vi "ArrDevMeasAction.vi"(7 "DevId":i32, 8 "error in (no error)":errorcluster caption="entrée d'erreur (pas d'erreur)", 9 "CurvePointIndex":i32, 10 "AllPointIndex":i32, 11 "Device In":refnum<class "MultiHarp150.lvclass"> caption="DNL_LabVIEW Object in") -> (0 "error out":errorcluster caption="sortie d'erreur", 1 "ArrDevDat":T1[](array[typedef]), 2 "ArrDevDatOut":dbl[][](array[numeric]), 3 "Device Out":refnum<class "MultiHarp150.lvclass"> caption="DNL_LabVIEW Object out", 5 "MeasOut":dbl[](array[numeric]))   [LabVIEW 2019, in "MultiHarp150.lvclass"]
uses:
  MultiHarp150.lvclass
  C:/Programmes Labview/LabscanV1A/DevicesClass/BaseDevice/BaseDevice.lvclass
  Experiment Class/ArrDevData.ctl
  MultiHarp150.lvclass/MultiHarp150.ctl
  <userlib>/MultiHarp150/T2Lib/MH_T2QMessage.ctl
  T2AcqStates.ctl
  <userlib>/GenProg/ReadValByRefI32.vi
  <vilib>/Utility/error.llb/Error Cluster From Error Code.vi
  <vilib>/ErrorRing/Error Ring.xnode
panel:
  out "TotalT":u32
  out "Desired LP":u32[](array[numeric])
  out "Loop DeltaT":u32[](array[numeric])
  out "RecRate":u32
  out "LoopPeriod":u32
  out "Record/ms":dbl
  in  "RecordsCnt":i64
  in  "OverRun":bool
  in  "Acq":bool
  out "Graph":refnum<vi>
  out "Dat":refnum<vi>
  in  "ViRef":refnum<vi>
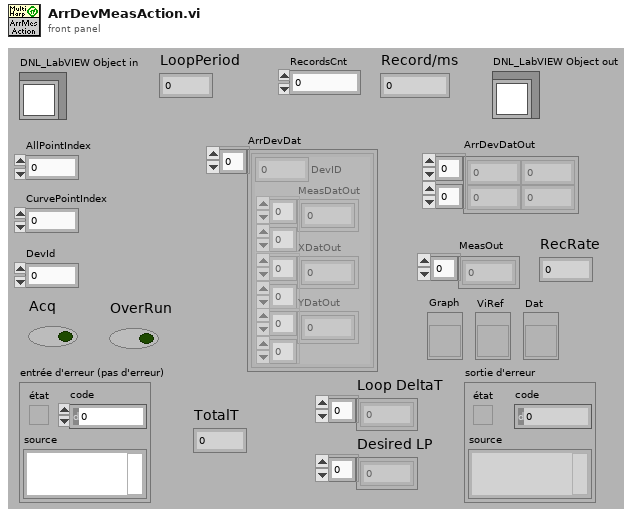
[diagram p1: front panel]
types:
  T1 = typedef "ArrDevData.ctl" = cluster{"MeasDatOut":dbl[][], "XDatOut":dbl[][], "YDatOut":dbl[][], "DevID":i32}
  T2 = cluster{"TotalCount":dbl, "HistRate (CPS)":dbl, "MaxTime":dbl}[]
  T3 = enum32{"Invalid", "Standard", "Closed", "Hidden", "Minimized", "Maximized"}
  T4 = typedef "T2AcqStates.ctl" = enum16{"checkStatus", "ReadFifo", "StopMeas", "Error", "End"}
  T5 = typedef "MH_T2QMessage.ctl" = cluster{"Message":string, "buffer":u32[], "Code":i32, "nactual":i32}
  T6 = typedef "MH_InputChannel_LS.ctl" = cluster{"Name":string, "Enable":bool, "Edge":i32, "Level":i32, "Offset":i32, "UseDeadTime":bool, "DeadTime":i32}
  T7 = typedef "MultiHarp150.lvclass/MultiHarp150_Func.ctl" = enum16{"ReadHistogram (Ph)", "ReadT2 (Ph)", "ReadT3 (Ph)", "ReadCount (Ph)"}
  T8 = cluster{dbl, "Resolution (ns)":dbl, "Histogram":u32[][]}
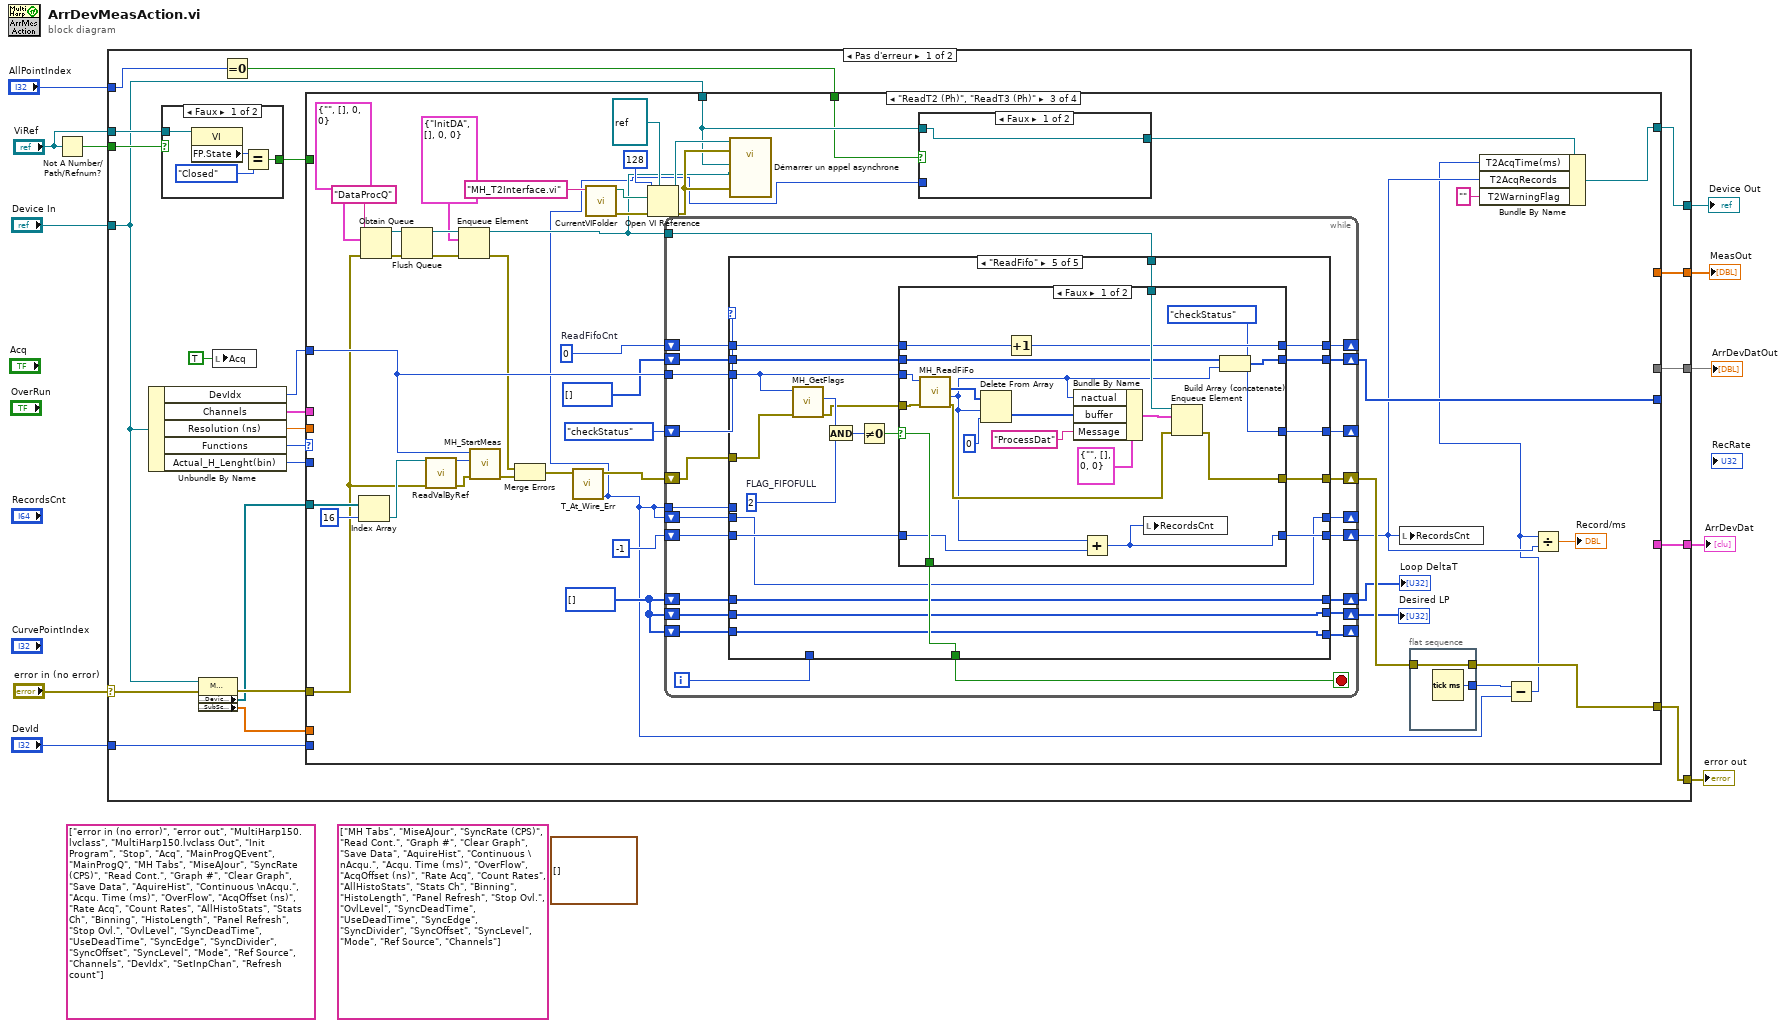
[diagram p0: block diagram]
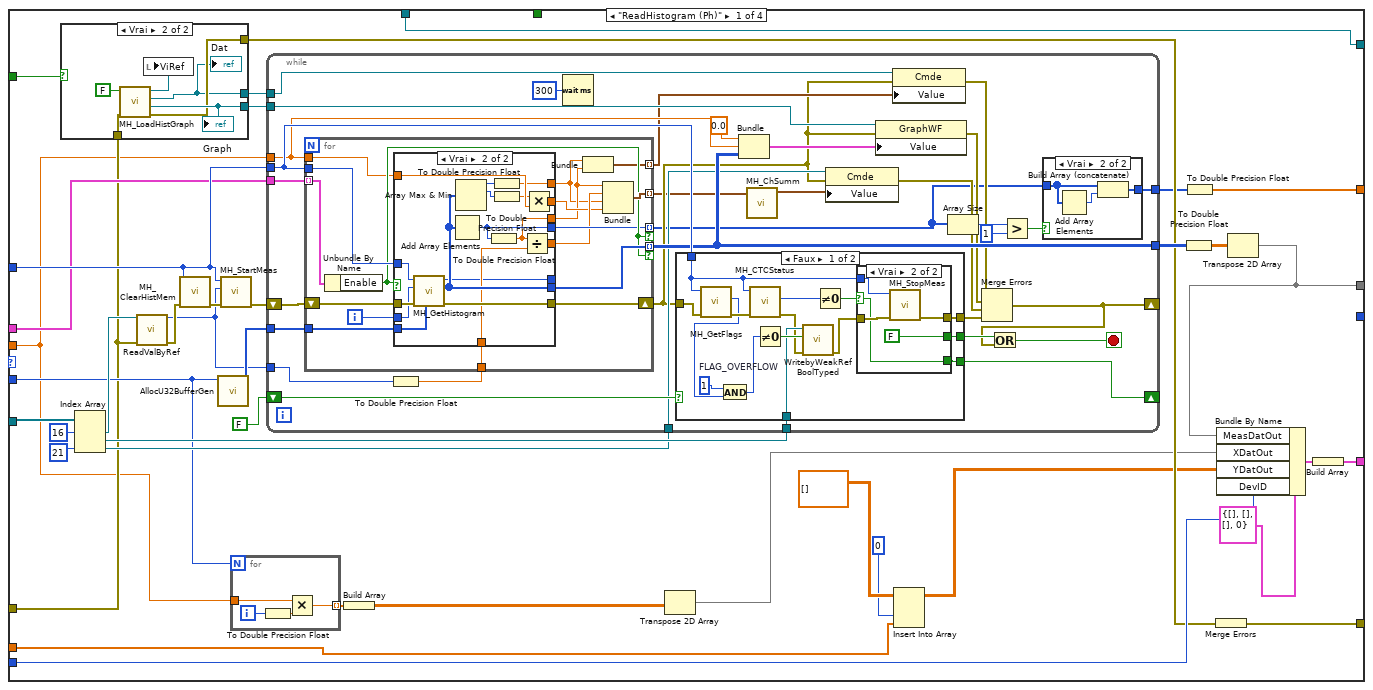
[diagram p3: hidden frame]
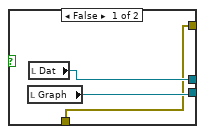
[diagram p4: hidden frame]
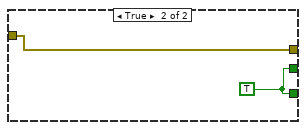
[diagram p7: hidden frame]
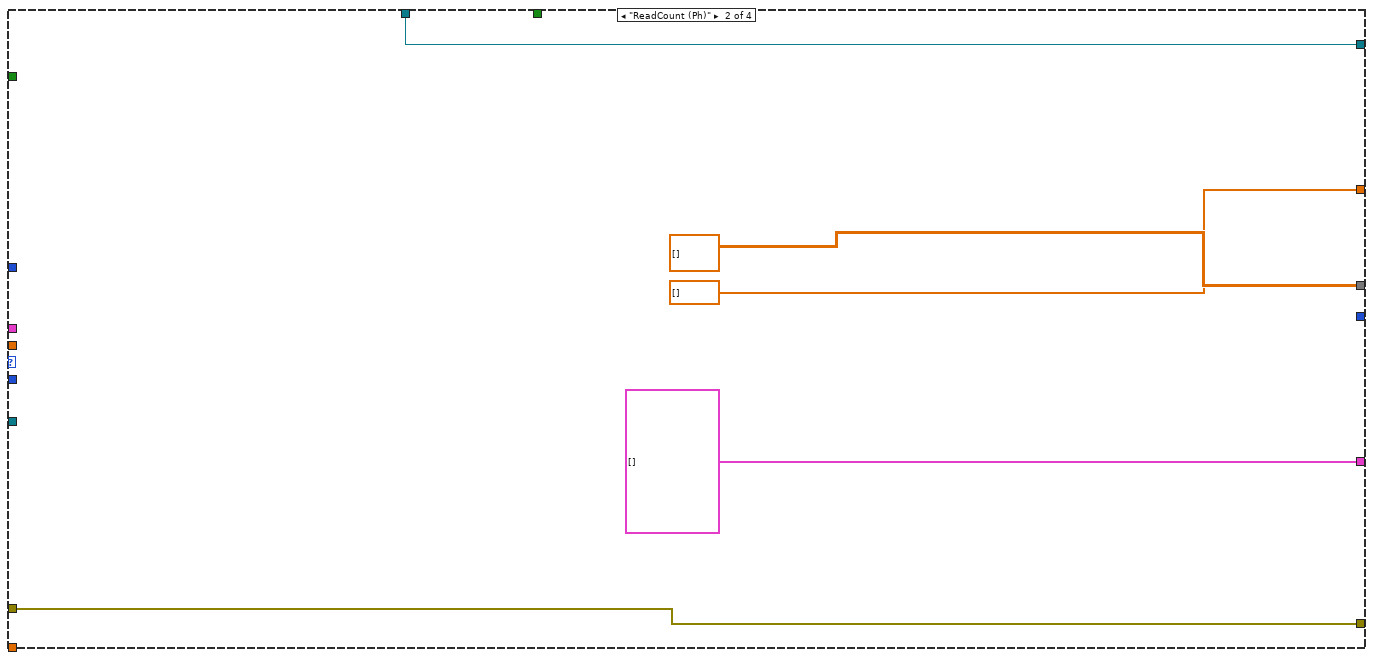
[diagram p9: hidden frame]
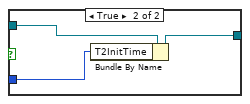
[diagram p10: hidden frame]
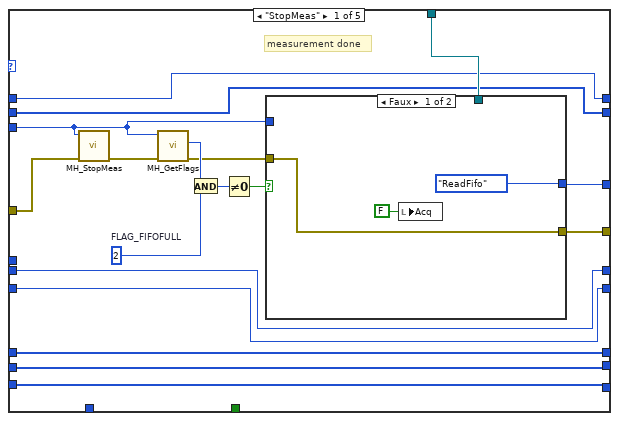
[diagram p11: hidden frame]
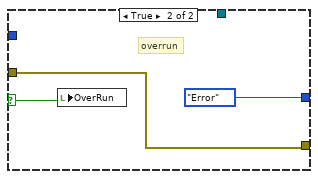
[diagram p12: hidden frame]
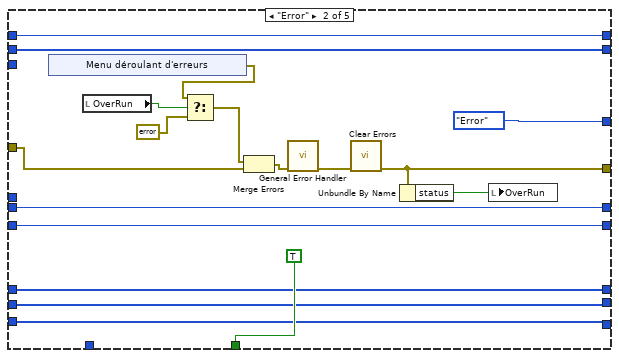
[diagram p13: hidden frame]
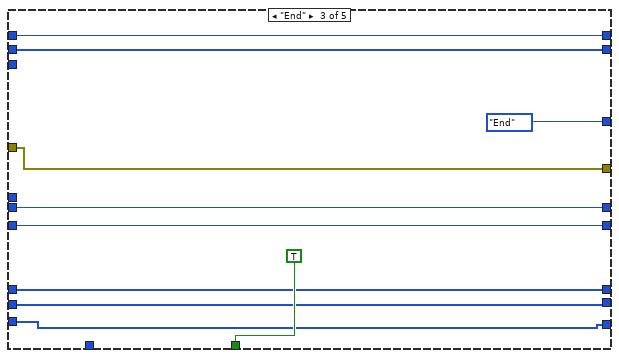
[diagram p14: hidden frame]
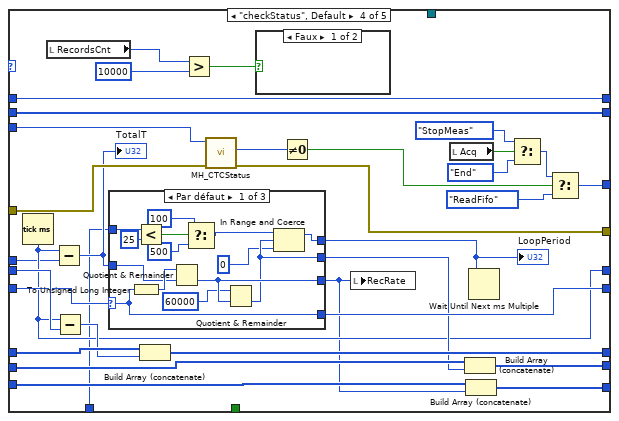
[diagram p15: hidden frame]
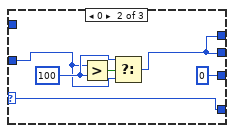
[diagram p16: hidden frame]
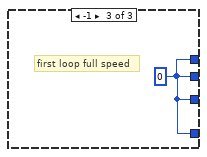
[diagram p17: hidden frame]
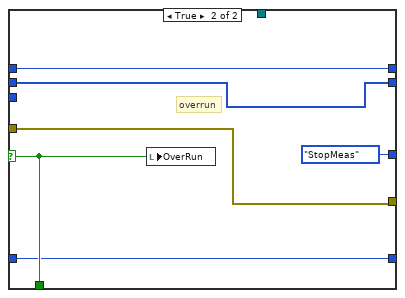
[diagram p19: hidden frame]
diagram:
  (unwired) string[][] [["MH Tabs"], ["MiseAJour"], ["SyncRate (CPS)"], ["Read Cont."], ["Graph #"], ["Clear Graph"], ["Save Data"], ["AquireHist"], ["Continuous \nAcqu."], ["Acqu. Time (ms)"], ["OverFlow"], ["AcqOffset (ns)"], ["Rate Acq"], ["Count Rates"], ["AllHistoStats"], ["Stats Ch"], ["Binning"], ["HistoLength"], ["Panel Refresh"], ["Stop Ovl."], ["OvlLevel"], ["SyncDeadTime"], ["UseDeadTime"], ["SyncEdge"], ["SyncDivider"], ["SyncOffset"], ["SyncLevel"], ["Mode"], ["Ref Source"], ["Channels"]] ("TabControls")
  (unwired) string[] ["error in (no error)", "error out", "MultiHarp150.lvclass", "MultiHarp150.lvclass Out", "Init Program", "Stop", "Acq", "MainProgQEvent", "MainProgQ", "MH Tabs", "MiseAJour", "SyncRate (CPS)", "Read Cont.", "Graph #", "Clear Graph", "Save Data", "AquireHist", "Continuous \nAcqu.", "Acqu. Time (ms)", "OverFlow", "AcqOffset (ns)", "Rate Acq", "Count Rates", "AllHistoStats", "Stats Ch", "Binning", "HistoLength", "Panel Refresh", "Stop Ovl.", "OvlLevel", "SyncDeadTime", "UseDeadTime", "SyncEdge", "SyncDivider", "SyncOffset", "SyncLevel", "Mode", "Ref Source", "Channels", "DevIdx", "SetInpChan", "Refresh count"] ("ControlsNames")
  (unwired) T2 [] ("AllHistoStats")
  n1 = Not A Number/Path/Refnum?(number/path/refnum="ViRef") -> (NaN/Path/Refnum?=w2:bool)
  n2 = case shown="Pas d'erreur" "error in (no error)" {
    selector: "error in (no error)" -> [w31 w431]
    tunnel: [w32 w431] -> w10
    tunnel: [w14 w430] -> w9
    tunnel: "Device In" -> [w15 w430]
    tunnel: "AllPointIndex" -> [w13 _]
    tunnel: [w28 dbl[] [] ("MeasOut 2")] -> w6
    tunnel: [w27 dbl[][] [] ("ArrDevDatOut 2")] -> w5
    tunnel: [w25 T1[] [] ("ArrDevDat 2")] -> w4
    tunnel: "DevId" -> [w26 _]
    tunnel: w2 -> [w17 _]
    tunnel: "ViRef" -> [w19 _]
    frame No Error {
      n3 = Unbundle By Name(w15) -> ("DevIdx"=w21:i32, "Channels"=w22:T6[], "Resolution (ns)"=w24:dbl, "Functions"=w33:T7, "Actual_H_Lenght(bin)"=w23:i32)
      n4 = case shown="Faux" w17 {
        selector: w17 -> [_ w38]
        tunnel: w19 -> [w37 _]
        tunnel: [w34 w38] -> w18
        frame False {
          n5 = property class="VI"(reference=w37) -> ("FP.State"=w36:T3)  [unwired: 1 in, 2 out]
          n6 = Equal?(x=w36, y=T3."Closed") -> (x = y?=w34:bool)
        }
        frame True {
        }
      }
      n7 = property class="MultiHarp150.lvclass"(reference=w15, error in=w31) -> (error out=w30:errorcluster, "Accessor:DeviceCtrl"=w29:refnum<vi>[], "Accessor:SubScanTable(y)"=w20:dbl[])  [unwired: 1 out]
      n8 = local write "Acq"(TRUE ("Acq")) -> ()
      n9 = Equal To 0?(x=w13) -> (x = 0?=w12:bool)
      n10 = case shown="\"ReadT2 (Ph)\", \"ReadT3 (Ph)\"" w33 {
        tunnel: [w65 w188 w217 w426] -> w32
        tunnel: w30 -> [w52 w188 w226 w426]
        tunnel: w29 -> [w53 _ w236 _]
        tunnel: [w69 dbl[] [] _ _] -> w28
        tunnel: [w46 dbl[][] [] _ _] -> w27
        tunnel: w26 -> [w74 _ _ _]
        tunnel: [w72 T1[] [] _ _] -> w25
        tunnel: w21 -> [w61 _ w231 _]
        tunnel: w24 -> [w45 _ _ _]
        tunnel: w23 -> [w55 _ _ _]
        tunnel: w22 -> [w56 _ _ _]
        tunnel: w20 -> [w54 _ _ _]
        tunnel: w18 -> [w43 _ _ _]
        tunnel: [_ _ w212 _] -> _
        tunnel: w15 -> [w39 w187 w194 w425]
        tunnel: [w39 w187 w201 w425] -> w14
        tunnel: w12 -> [_ _ w193 _]
        frame "ReadHistogram (Ph)" {
          n11 = case shown="Vrai" w43 {
            tunnel: [w80 w86] -> w63
            tunnel: [w78 w85] -> w62
            tunnel: w52 -> [w78 w84]
            tunnel: [w79 w83] -> w44
            frame False {
              n12 = local read "Graph"() -> (w80:refnum<vi>)
              n13 = local read "Dat"() -> (w79:refnum<vi>)
            }
            frame True {
              n14 = call <userlib>:"MH_LoadHistGraph.vi"("ErrIn(No Err)"=w84, "Rate Mode"=FALSE) -> ("ErrOut"=w85:errorcluster, "Graph"=w86:refnum<vi>, "Dat"=w83:refnum<vi>, "ViRef"=w82:refnum<vi>)  [unwired: 4 in, 2 out]
              "Dat" <- w83
              "Graph" <- w86
              n15 = local write "ViRef"(w82) -> ()
            }
          }
          n16 = Index Array(array=w53, index #1=16 ("indice"), index #3=21 ("indice")) -> (element #1=w76:refnum<vi>, element #2=w66:refnum<vi>, element #3=w57:refnum<vi>)  [unwired: 1 in]
          n17 = call-poly <userlib>:"ReadValByRef.vi"("Control Ref"=w76, "error in"=w52) -> ("Valeur"=w40:i32, "error out"=w67:errorcluster)  [unwired: 12 in]
          n18 = call <userlib>:"MH_ClearHistMem.vi"("error in (no error)"=w67, "devidx"=w61) -> ("error out"=w68:errorcluster)  [unwired: 8 in, 1 out]
          n19 = call <userlib>:"AllocU32BufferGen.vi"("BuffLength"=w55) -> ("Buffer"=w71:u32[])  [unwired: 10 in]
          n20 = call <userlib>:"MH_StartMeas.vi"("error in (no error)"=w68, "tacq"=w40, "devidx"=w61) -> ("error out"=w70:errorcluster)  [unwired: 7 in, 1 out]
          n21 = for {
            N: w55 -> [_]
            tunnel: w45 -> [w90]
            tunnel: [w87] -> w42 mode=indexing
            i -> [w89]
            n22 = To Double Precision Float(number=w89) -> (double precision float=w88:dbl)
            n23 = Multiply(x=w90, y=w88) -> (x*y=w87:dbl)
          }
          n24 = while {
            tunnel: w56 -> [w106]
            tunnel: [w117] -> w64
            tunnel: w61 -> [w120]
            shift-right: [w111] -> _
            shift-left: w70 -> [w122]
            tunnel: w71 -> [w123]
            tunnel: w66 -> [w119]
            tunnel: w45 -> [w105]
            tunnel: w63 -> [w115]
            shift-right: [w110] -> _
            shift-left: FALSE -> [w109]
            tunnel: [w95] -> w58
            tunnel: w57 -> [w108]
            tunnel: w40 -> [w107]
            tunnel: w44 -> [w104]
            stop <- w113 stop-if-true
            n25 = To Double Precision Float(number=w107) -> (double precision float=w93:dbl)
            n26 = for {
              tunnel: w123 -> [w168]
              tunnel: w120 -> [w167]
              tunnel: w106 -> [w164] mode=indexing
              shift-right: [w165] -> w101
              shift-left: w122 -> [w166]
              tunnel: [w163] -> w117 mode=indexing if=w161
              tunnel: [w159] -> w96 mode=indexing if=w161
              tunnel: w105 -> [w157]
              tunnel: [w162] -> w91 mode=indexing
              tunnel: w93 -> [w160]
              tunnel: [w156] -> w103 mode=indexing
              i -> [w154]
              n27 = Unbundle By Name(w164) -> ("Enable"=w161:bool)
              n28 = case shown="Vrai" w161 {
                tunnel: w168 -> [_ w186]
                tunnel: w167 -> [_ w175]
                tunnel: [_ w182] -> w163
                tunnel: w166 -> [w169 w185]
                tunnel: [w169 w184] -> w165
                tunnel: w154 -> [_ w183]
                tunnel: [_ w178] -> w159
                tunnel: w157 -> [_ w180]
                tunnel: [_ w179] -> w155
                tunnel: w160 -> [_ w177]
                tunnel: [_ w176] -> w158
                tunnel: [_ w174] -> _
                tunnel: [_ w173] -> w153
                tunnel: [_ w171] -> w152
                frame False {
                }
                frame True {
                  n29 = call <userlib>:"MH_GetHistogram.vi"("Chcount"=w186, "error in (no error)"=w185, "channel"=w183, "devidx"=w175) -> ("error out"=w184:errorcluster, "Histogram"=w182:u32[], "return type"=w174:i32)  [unwired: 5 in]
                  n30 = Add Array Elements(numeric array=w182) -> (sum=w178:u32)
                  n31 = Array Max & Min(array=w182) -> (max value=w172:u32, max index (indices)=w181:i32)  [unwired: 2 out]
                  n32 = To Double Precision Float(number=w178) -> (double precision float=w173:dbl)
                  n33 = To Double Precision Float(number=w172) -> (double precision float=w171:dbl)
                  n34 = To Double Precision Float(number=w181) -> (double precision float=w170:dbl)
                  n35 = Divide(x=w173, y=w177) -> (x/y=w176:dbl)
                  n36 = Multiply(x=w170, y=w180) -> (x*y=w179:dbl)
                }
              }
              n37 = Bundle(w152, w153) -> (w156:cluster{dbl, dbl})  [unwired: 1 in]
              n38 = Bundle(w153, w158, w152, w155) -> (w162:cluster{dbl, dbl, dbl, dbl})  [unwired: 1 in]
            }
            n39 = Wait (ms)(milliseconds to wait=u32 300 ("attente (ms)")) -> ()  [unwired: 1 out]
            n40 = case shown="Faux" w109 {
              tunnel: w101 -> [w136 w151]
              tunnel: [w131 w150] -> w121
              tunnel: w120 -> [w135 _]
              tunnel: w119 -> [w137 _]
              tunnel: [w133 w151] -> w112
              tunnel: [w130 w150] -> w110
              frame False {
                w140 = 1  # FLAG_OVERFLOW
                n41 = call <userlib>:"MH_GetFlags.vi"("error in (no error)"=w136, "devidx"=w135) -> ("error out"=w142:errorcluster, "flags"=w139:i32)  [unwired: 7 in, 1 out]
                n42 = And(x=w140, y=w139) -> (x .and. y?=w141:i32)
                n43 = call <userlib>:"MH_CTCStatus.vi"("error in (no error)"=w142, "devidx"=w135) -> ("error out"=w129:errorcluster, "ctcstatus"=w134:i32)  [unwired: 7 in, 1 out]
                n44 = Not Equal To 0?(x=w141) -> (x != 0?=w138:bool)
                n45 = call <userlib>:"WritebyWeakRefBoolTyped.vi"("error in"=w129, "Valeur"=w138, "Control Ref"=w137) -> ("error out"=w128:errorcluster)  [unwired: 8 in]
                n46 = Not Equal To 0?(x=w134) -> (x != 0?=w132:bool)
                n47 = case shown="Vrai" w132 {
                  selector: w132 -> [w143 w145]
                  tunnel: w135 -> [_ w147]
                  tunnel: w128 -> [w144 w149]
                  tunnel: [w144 w148] -> w133
                  tunnel: [w143 FALSE] -> w131
                  tunnel: [w143 w145] -> w130
                  frame False {
                  }
                  frame True {
                    n48 = call <userlib>:"MH_StopMeas.vi"("error in (no error)"=w149, "devidx"=w147) -> ("error out"=w148:errorcluster)  [unwired: 8 in, 1 out]
                  }
                }
              }
              frame True {
                w150 = TRUE
              }
            }
            n49 = Bundle(0.0, "Resolution (ns)"=w105, "Histogram"=w117) -> (w114:T8)  [unwired: 1 in]
            n50 = call <userlib>:"MH_ChSumm.vi"("HistDat"=w91) -> ("HistDat Out"=w92:cluster{dbl, dbl, dbl, dbl}[])  [unwired: 10 in]
            n51 = property class="Cmde"(reference=w108, error in=w101, "Value"=w92) -> (error out=w100:errorcluster)  [unwired: 1 out]
            n52 = property class="GraphWF"(reference=w115, error in=w101, "Value"=w114) -> (error out=w99:errorcluster)  [unwired: 1 out]
            n53 = property class="Cmde"(reference=w104, error in=w101, "Value"=w103) -> (error out=w102:errorcluster)  [unwired: 1 out]
            n54 = Array Size(array=w96) -> (size(s)=w98:i32)
            n55 = Merge Errors(w102, w99, w100, w112) -> (w111:errorcluster)
            n56 = Or(x=w121, y=w111) -> (x .or. y?=w113:bool)
            n57 = Greater?(x=w98, y=1) -> (0:w94:bool)
            n58 = case shown="Vrai" w94 {
              tunnel: w96 -> [w124 w126]
              tunnel: [w124 w125] -> w95
              frame False {
              }
              frame True {
                n59 = Add Array Elements(numeric array=w126) -> (sum=w127:u32)
                n60 = Build Array (concatenate)(w126, w127) -> (w125:u32[])
              }
            }
          }
          n61 = Build Array(w42) -> (w41:dbl[][])
          n62 = Transpose 2D Array(2D array=w41) -> (transposed array=w48:dbl[][])
          n63 = Insert Into Array(array=dbl[][] [] ("tableau"), index (col)=0 ("indice désactivé (col)"), new element=w54) -> (w51:dbl[][])  [unwired: 1 in]
          n64 = To Double Precision Float(number=w64) -> (double precision float=w47:dbl[][])
          n65 = To Double Precision Float(number=w58) -> (double precision float=w69:dbl[])
          n66 = Merge Errors(w62) -> (w65:errorcluster)
          n67 = Transpose 2D Array(2D array=w47) -> (transposed array=w46:dbl[][])
          n68 = Bundle By Name(cluster=T1 {"MeasDatOut"=[], "XDatOut"=[], "YDatOut"=[], "DevID"=0} ("cluster de sortie"), "MeasDatOut"=w46, "XDatOut"=w48, "YDatOut"=w51, "DevID"=w74) -> (w73:T1)
          n69 = Build Array(w73) -> (w72:T1[])
        }
        frame "ReadCount (Ph)" {
        }
        frame "ReadT2 (Ph)", "ReadT3 (Ph)" {
          w210 = u32[] []
          w221 = u32 0  # ReadFifoCnt
          n70 = Index Array(array=w236, index=16 ("indice")) -> (element=w235:refnum<vi>)
          n71 = Obtain Queue(name (unnamed)="DataProcQ", element data type=T5 {"Message"="", "buffer"=[], "Code"=0, "nactual"=0} ("ClassQueue"), error in (no error)=w226) -> (queue out=w230:refnum<queue>, error out=w229:errorcluster)  [unwired: 2 in, 1 out]
          n72 = Flush Queue(queue=w230, error in (no error)=w229) -> (queue out=w225:refnum<queue>, error out=w224:errorcluster)  [unwired: 1 out]
          n73 = call-poly <userlib>:"ReadValByRef.vi"("Control Ref"=w235, "error in"=w226) -> ("Valeur"=w234:i32, "error out"=w233:errorcluster)  [unwired: 12 in]
          n74 = Enqueue Element(queue=w225, element=T5 {"Message"="InitDA", "buffer"=[], "Code"=0, "nactual"=0} ("élément"), error in (no error)=w224) -> (queue out=w202:refnum<queue>, error out=w223:errorcluster)  [unwired: 1 in, 1 out]
          n75 = call <userlib>:"MH_StartMeas.vi"("error in (no error)"=w233, "tacq"=w234, "devidx"=w231) -> ("error out"=w232:errorcluster)  [unwired: 7 in, 1 out]
          n76 = Merge Errors(w223, w232) -> (w197:errorcluster)
          n77 = call <userlib>:"T_At_Wire_Err.vi"("error in (no error)"=w197) -> ("Clock(ms)"=w192:u32, "error out"=w196:errorcluster)  [unwired: 8 in, 1 out]
          n78 = call <userlib>:"CurrentVIFolder.vi"("NomFichier"="MH_T2Interface.vi" ("nom ou chemin relatif")) -> ("error out"=w205:errorcluster, "Chemin"=w204:path)  [unwired: 8 in, 1 out]
          n79 = Open VI Reference(type specifier VI Refnum (for type only)=refnum<vi> refnum ("spécificateur de type du refnum de VI (pour type seulement)"), vi path=w204, options=128, error in (no error)=w205) -> (vi reference=w203:refnum<vi>, error out=w208:errorcluster)  [unwired: 2 in]
          n80 = while {
            shift-right: [w266] -> w218
            shift-left: w196 -> [w258]
            tunnel: w231 -> [w262]
            tunnel: w202 -> [w264]
            shift-right: [w260] -> _
            shift-left: w221 -> [w261]
            shift-right: [w257] -> _
            shift-left: T2AcqStates."checkStatus" -> [w259]
            shift-right: [w256] -> w200
            shift-left: i64 -1 ("RecordsCnt") -> [w255]
            shift-right: [w251] -> w214
            shift-left: w210 -> [w252]
            shift-right: [w253] -> _
            shift-left: w192 -> [w254]
            shift-right: [w249] -> w212
            shift-left: i32[] [] -> [w250]
            shift-right: [w247] -> w211
            shift-left: w210 -> [w248]
            tunnel: w192 -> [w246]
            shift-right: [w244] -> _
            shift-left: w210 -> [w245]
            i -> [w263]
            stop <- w265 stop-if-true
            n81 = case shown="\"ReadFifo\"" w259 {
              tunnel: w262 -> [w277 _ _ w354 w393]
              tunnel: w258 -> [w276 w303 w323 w355 w395]
              tunnel: [w279 w298 w323 w345 w391] -> w266
              tunnel: [_ TRUE TRUE _ w390] -> w265
              tunnel: w264 -> [w278 _ _ _ w389]
              tunnel: w263 -> [_ _ _ w324 _]
              tunnel: w261 -> [w274 w306 w320 w352 w388]
              tunnel: [w274 w306 w320 w352 w387] -> w260
              tunnel: [w273 T2AcqStates."Error" T2AcqStates."End" w351 w386] -> w257
              tunnel: [w272 w296 w319 w340 w385] -> w256
              tunnel: w255 -> [w272 w296 w319 w341 w384]
              tunnel: w254 -> [w271 w295 w318 w344 w383]
              tunnel: [w271 w295 w318 w332 w383] -> w253
              tunnel: w252 -> [w270 w294 w317 w339 w382]
              tunnel: [w270 w294 w317 w337 w382] -> w251
              tunnel: w250 -> [w269 w293 w316 w335 w380]
              tunnel: [w269 w293 w316 w335 w381] -> w249
              tunnel: w248 -> [w268 w292 w315 w334 w379]
              tunnel: [w268 w292 w315 w329 w379] -> w247
              tunnel: w246 -> [_ _ _ w331 _]
              tunnel: w245 -> [w267 w291 w314 w328 w378]
              tunnel: [w267 w291 w314 w326 w378] -> w244
              frame "StopMeas" {
                w283 = 2  # FLAG_FIFOFULL
                # "measurement done"
                n82 = call <userlib>:"MH_StopMeas.vi"("error in (no error)"=w276, "devidx"=w277) -> ("error out"=w275:errorcluster)  [unwired: 8 in, 1 out]
                n83 = call <userlib>:"MH_GetFlags.vi"("error in (no error)"=w275, "devidx"=w277) -> ("error out"=w280:errorcluster, "flags"=w282:i32)  [unwired: 7 in, 1 out]
                n84 = And(x=w282, y=w283) -> (x .and. y?=w284:i32)
                n85 = Not Equal To 0?(x=w284) -> (x != 0?=w281:bool)
                n86 = case shown="Faux" w281 {
                  selector: w281 -> [_ w288]
                  tunnel: w277 -> [_ _]
                  tunnel: w280 -> [w286 w290]
                  tunnel: [w286 w290] -> w279
                  tunnel: w278 -> [_ _]
                  tunnel: [T2AcqStates."ReadFifo" T2AcqStates."Error"] -> w273
                  frame False {
                    n87 = local write "Acq"(FALSE ("Acq")) -> ()
                  }
                  frame True {
                    # "overrun"
                    n88 = local write "OverRun"(w288) -> ()
                  }
                }
              }
              frame "Error" {
                n89 = xnode "Menu déroulant d'erreurs"() -> ("sortie d'erreur"=w299:errorcluster)
                n90 = local read "OverRun"() -> (w304:bool)
                n91 = Select(t=w299, s=w304, f=errorcluster {"status"=FALSE, "code"=0, "source"=""} ("cas vrai")) -> (s? t:f=w300:errorcluster)
                n92 = Merge Errors(w300, w303) -> (w301:errorcluster)
                n93 = call <vilib>:"General Error Handler.vi"("error in (no error)"=w301) -> ("error out"=w305:errorcluster)  [unwired: 10 in, 4 out]
                n94 = call <vilib>:"Clear Errors.vi"("error in (no error)"=w305) -> ("error out"=w298:errorcluster)  [unwired: 5 in, 1 out]
                n95 = Unbundle By Name(w298) -> ("status"=w297:bool)
                n96 = local write "OverRun"(w297) -> ()
              }
              frame "End" {
              }
              frame "checkStatus", Default {
                n97 = Tick Count (ms)() -> (millisecond timer value=w332:u32)
                n98 = local read "RecordsCnt"() -> (w343:i64)
                n99 = Subtract(x=w332, y=w331) -> (x-y=w330:u32)
                "TotalT" <- w330
                n100 = Subtract(x=w332, y=w344) -> (x-y=w338:u32)
                n101 = case shown="Par défaut" w341 {
                  selector: w341 -> [w368 w373 _]
                  tunnel: w330 -> [w366 w372 _]
                  tunnel: [w370 u32 0 w377] -> w327
                  tunnel: [w365 w371 w377] -> w333
                  tunnel: [w368 w373 w377] -> w340
                  tunnel: [w363 w371 w377] -> w325
                  tunnel: w324 -> [w362 _ _]
                  frame Default {
                    n102 = To Unsigned Long Integer(number=w368) -> (unsigned 32bit integer=w367:u32)
                    n103 = Less?(x=w362, y=25) -> (x < y?=w360:bool)
                    n104 = Quotient & Remainder(x=w367, y=w366) -> (floor(x/y)=w370:u32)  [unwired: 1 out]
                    n105 = Select(t=u32 100 ("cas vrai"), s=w360, f=u32 500 ("limite supérieure")) -> (s? t:f=w357:u32)
                    n106 = Quotient & Remainder(x=u32 60000, y=w370) -> (floor(x/y)=w365:u32)  [unwired: 1 out]
                    n107 = In Range and Coerce(upper limit=w357, x=w365, lower limit=u32 0 ("limite inférieure")) -> (coerced(x)=w363:u32)  [unwired: 1 out]
                  }
                  frame 0 {
                    w374 = u32 100 ("y")
                    n108 = Greater?(x=w372, y=w374) -> (0:w375:bool)
                    n109 = Select(t=w374, s=w375, f=w372) -> (s? t:f=w371:u32)
                  }
                  frame -1 {
                    w377 = u32 0
                    # "first loop full speed"
                  }
                }
                "LoopPeriod" <- w325
                n110 = Build Array (concatenate)(w339, w338) -> (w337:u32[])
                n111 = Greater?(x=w343, y=10000) -> (0:w342:bool)
                n112 = call <userlib>:"MH_CTCStatus.vi"("error in (no error)"=w355, "devidx"=w354) -> ("error out"=w345:errorcluster, "ctcstatus"=w356:i32)  [unwired: 7 in, 1 out]
                n113 = case shown="Faux" w342 {
                  frame False {
                  }
                  frame True {
                  }
                }
                n114 = Not Equal To 0?(x=w356) -> (x != 0?=w336:bool)
                n115 = local write "RecRate"(w327) -> ()
                n116 = local read "Acq"() -> (w349:bool)
                n117 = Build Array (concatenate)(w334, w333) -> (w329:u32[])
                n118 = Build Array (concatenate)(w328, w327) -> (w326:u32[])
                n119 = Wait Until Next ms Multiple(millisecond multiple=w325) -> ()  [unwired: 1 out]
                n120 = Select(t=T2AcqStates."StopMeas", s=w349, f=T2AcqStates."End") -> (s? t:f=w347:T4)
                n121 = Select(t=w347, s=w336, f=T2AcqStates."ReadFifo") -> (s? t:f=w351:T4)
              }
              frame "ReadFifo" {
                w397 = 2  # FLAG_FIFOFULL
                n122 = call <userlib>:"MH_GetFlags.vi"("error in (no error)"=w395, "devidx"=w393) -> ("error out"=w392:errorcluster, "flags"=w396:i32)  [unwired: 7 in, 1 out]
                n123 = And(x=w396, y=w397) -> (x .and. y?=w398:i32)
                n124 = Not Equal To 0?(x=w398) -> (x != 0?=w394:bool)
                n125 = case shown="Faux" w394 {
                  selector: w394 -> [w416 w421]
                  tunnel: w393 -> [w418 _]
                  tunnel: w392 -> [w417 w422]
                  tunnel: [w414 w422] -> w391
                  tunnel: [w416 w421] -> w390
                  tunnel: w389 -> [w415 _]
                  tunnel: w388 -> [w413 w424]
                  tunnel: [w412 w424] -> w387
                  tunnel: [T2AcqStates."checkStatus" T2AcqStates."StopMeas"] -> w386
                  tunnel: [w403 w420] -> w385
                  tunnel: w384 -> [w409 w420]
                  tunnel: [w405 w419] -> w381
                  tunnel: w380 -> [w404 w419]
                  frame False {
                    n126 = call <userlib>:"MH_ReadFiFo.vi"("error in (no error)"=w417, "devidx"=w418) -> ("error out"=w410:errorcluster, "nactual"=w399:i32, "buffer"=w402:u32[])  [unwired: 6 in, 1 out]
                    n127 = Delete From Array(array=w402, length=w399, index=0 ("indice")) -> (deleted portion=w401:u32[])  [unwired: 1 out]
                    n128 = Increment(x=w413) -> (x+1=w412:u32)
                    n129 = Bundle By Name(cluster=T5 {"Message"="", "buffer"=[], "Code"=0, "nactual"=0} ("ClassQueue"), "nactual"=w399, "buffer"=w401, "Message"="ProcessDat") -> (w408:T5)
                    n130 = Add(x=w399, y=w409) -> (x+y=w403:i64)
                    n131 = local write "RecordsCnt"(w403) -> ()
                    n132 = Enqueue Element(queue=w415, element=w408, error in (no error)=w410) -> (error out=w414:errorcluster)  [unwired: 1 in, 2 out]
                    n133 = Build Array (concatenate)(w404, w399) -> (w405:i32[])
                  }
                  frame True {
                    # "overrun"
                    n134 = local write "OverRun"(w421) -> ()
                  }
                }
              }
            }
          }
          "Loop DeltaT" <- w214
          "Desired LP" <- w211
          n135 = call-by-ref "Démarrer un appel asynchrone"(reference=w203, error in=w208, 8:"error in (no error)"=w208, "DataProcessQ"=w202, "Device In"=w194) -> ()  [unwired: 8 in, 3 out]
          n136 = case shown="Faux" w193 {
            tunnel: [w238 w240] -> w195
            tunnel: w194 -> [w238 w241]
            tunnel: w192 -> [_ w239]
            frame False {
            }
            frame True {
              n137 = Bundle By Name(cluster=w241, "T2InitTime"=w239) -> (w240:refnum<class "MultiHarp150.lvclass">)
            }
          }
          n138 = local write "RecordsCnt"(w200) -> ()
          n139 = flat-sequence {
            tunnel: [w243] -> w216
            tunnel: w218 -> [w242]
            tunnel: [w242] -> w217
            frame #0 {
              n140 = Tick Count (ms)() -> (millisecond timer value=w243:u32)
            }
          }
          n141 = Subtract(x=w216, y=w192) -> (x-y=w199:u32)
          n142 = Bundle By Name(cluster=w195, "T2AcqTime(ms)"=w199, "T2AcqRecords"=w200, "T2WarningFlag"="") -> (w201:refnum<class "MultiHarp150.lvclass">)
          n143 = Divide(x=w199, y=w200) -> (x/y=→"Record/ms":dbl)
        }
        frame Default {
        }
      }
    }
    frame Error {
    }
  }
  "error out" <- w10
  "Device Out" <- w9
  "ArrDevDatOut" <- w5
  "ArrDevDat" <- w4
  "MeasOut" <- w6
